vi "Power Qualtiy - 1.vi"() -> ()   [LabVIEW 2015]
uses:
  <vilib>/addons/Electrical Power/PQ/NI_EP_Power Quality.lvlib
  <vilib>/addons/Electrical Power/PQ/Aggregation/Custom Aggregation (DBL).vi
  <vilib>/addons/Electrical Power/PQ/Power_Energy/Power Values (Single Line).vi
  <vilib>/addons/Electrical Power/Basic/NI_EP_Basic.lvlib
  <vilib>/addons/Electrical Power/Basic/Measurement/Fundamental Vector (1 Channel).vi
  <vilib>/addons/Electrical Power/PQ/Common/Classes/System Info/EP System Info.lvclass
  <vilib>/addons/Electrical Power/PQ/Common/Controls/ep_AI Data Channel.ctl
  <vilib>/addons/Electrical Power/PQ/Common/Controls/ep_Aggregation Settings.ctl
  <vilib>/addons/Electrical Power/PQ/Common/Controls/ep_Event Type.ctl
  <vilib>/addons/Electrical Power/PQ/Common/Controls/ep_Phase.ctl
panel:
  out "system info out":refnum<class "EP System Info.lvclass">
  out "Pinst (Voltage Flicker Values)":waveform(dbl)[](array[waveform])
  out "rapid voltage changes events":T2(array[cluster])
  out "voltage flags":bool[](array[boolean])
  out "voltage events":T4(array[cluster])
  in  "events settings":T5={"swell threshold [%]"=110.0, "dip threshold [%]"=90.0, "interruption threshold [%]"=1.0, "hysteresis [%]"=2.0}
  out "THD [%]":dbl[](array[numeric])
  out "energy values":T6
  out "total power values":T7
  out "aggregated data timestamp":timestamp
  out "aggregated maximum value":dbl
  out "aggregated averaged/RMS value":dbl
  out "aggregated minimum value":dbl
  in  "data timestamp":timestamp
  in  "aggregation settings":T8={"interval"=1, "interval unit"=enum."Runs", "synchronization of intervals"=enum."Not synchronized", "algorithm"=enum."Average"}
  out "spectra":T10(array[cluster])
  # "System Settings"
  # "Power & Energy"
  # "Voltage"
  # "Current"
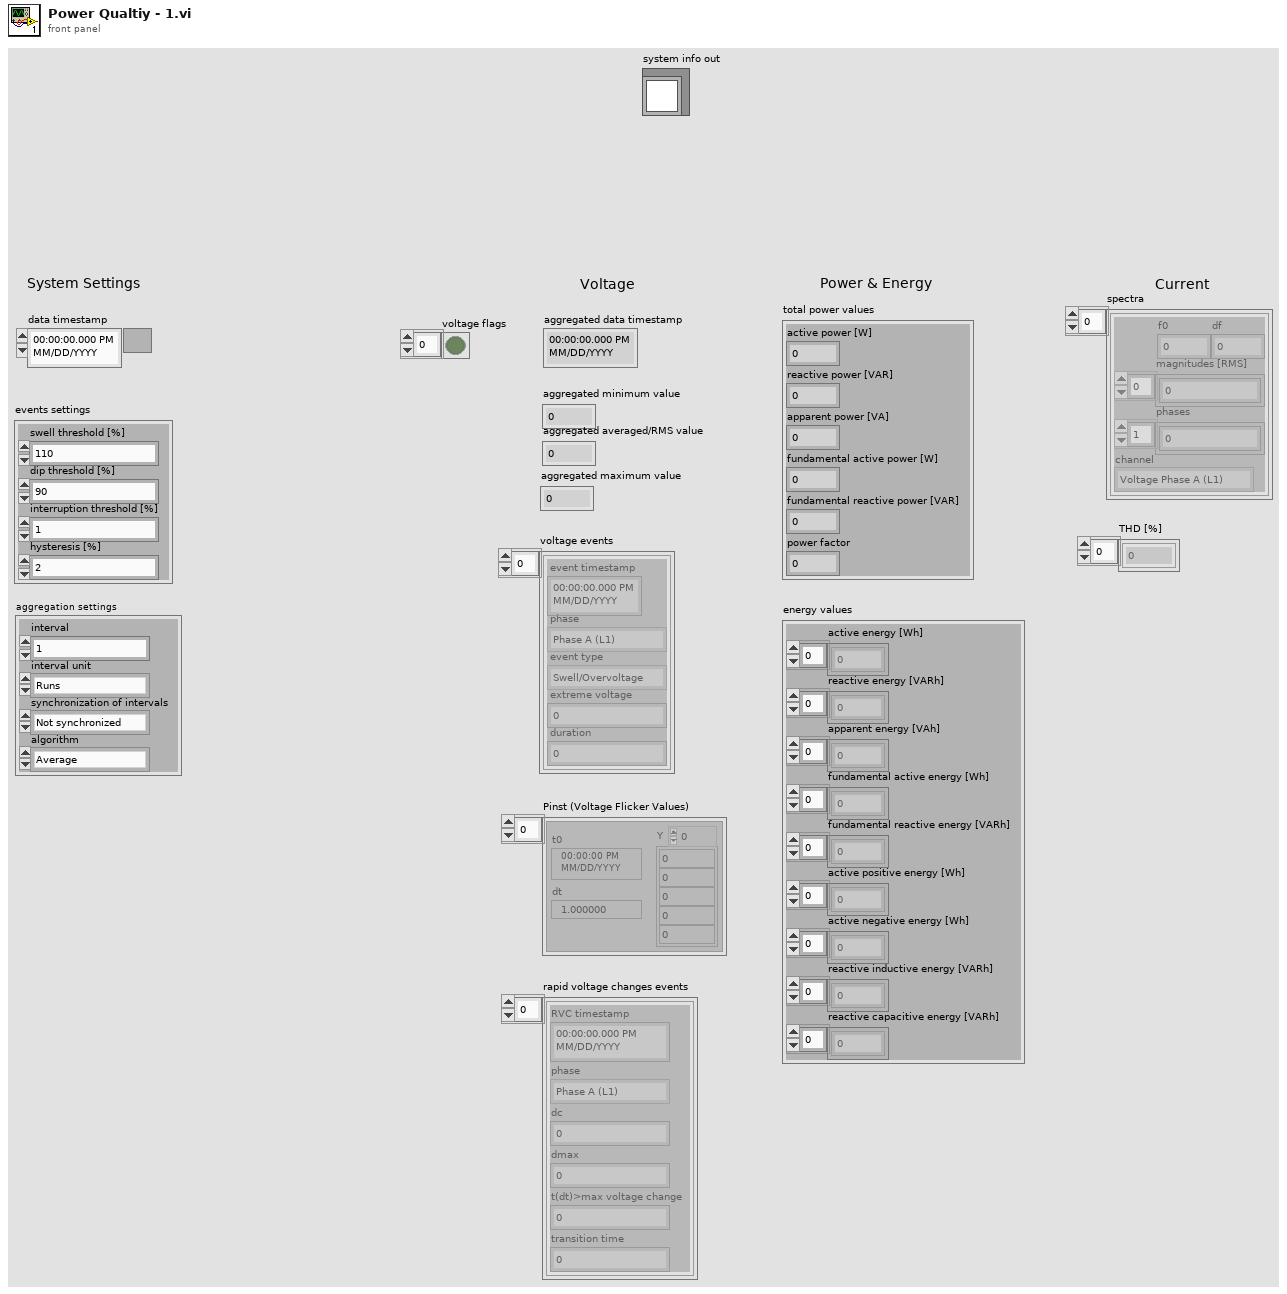
[diagram p1: front panel]
types:
  T1 = typedef "NI_EP_Power Quality.lvlib/ep_Phase.ctl" = enum16{"Phase A (L1)", "Phase B (L2)", "Phase C (L3)", "Phase N", "~3 Phases"}
  T2 = cluster{"RVC timestamp":timestamp, "phase":T1, "dc":dbl, "dmax":dbl, "t(dt)>max voltage change":dbl, "transition time":dbl}[]
  T3 = typedef "NI_EP_Power Quality.lvlib/ep_Event Type.ctl" = enum16{"Swell/Overvoltage", "Dip/Undervoltage", "Interruption"}
  T4 = cluster{"event timestamp":timestamp, "phase":T1, "event type":T3, "extreme voltage":dbl, "duration":dbl}[]
  T5 = cluster{"swell threshold [%]":dbl, "dip threshold [%]":dbl, "interruption threshold [%]":dbl, "hysteresis [%]":dbl}
  T6 = cluster{"active energy [Wh]":dbl[], "reactive energy [VARh]":dbl[], "apparent energy [VAh]":dbl[], "fundamental active energy [Wh]":dbl[], "fundamental reactive energy [VARh]":dbl[], "active positive energy [Wh]":dbl[], "active negative energy [Wh]":dbl[], "reactive inductive energy [VARh]":dbl[], "reactive capacitive energy [VARh]":dbl[]}
  T7 = cluster{"active power [W]":dbl, "reactive power [VAR]":dbl, "apparent power [VA]":dbl, "fundamental active power [W]":dbl, "fundamental reactive power [VAR]":dbl, "power factor":dbl}
  T8 = typedef "NI_EP_Power Quality.lvlib/ep_Aggregation Settings.ctl" = cluster{"interval":u32, "interval unit":enum16{"Runs", "Seconds", "Minutes", "Hours", "Days", "Weeks"}, "synchronization of intervals":enum16{"Not synchronized", "Interval rounded"}, "algorithm":enum16{"Average", "RMS"}}
  T9 = typedef "NI_EP_Power Quality.lvlib/ep_AI Data Channel.ctl" = enum16{"Voltage Phase A (L1)", "Voltage Phase B (L2)", "Voltage Phase C (L3)", "Voltage Phase N (Neutral)", "Current Phase A (L1)", "Current Phase B (L2)", "Current Phase C (L3)", "Current Phase N (Neutral)"}
  T10 = cluster{"f0":dbl, "df":dbl, "magnitudes [RMS]":dbl[], "phases":dbl[], "channel":T9}[]
  T11 = cluster{"timestamps":timestamp[], "RMS values":dbl[]}[]
  T12 = cluster{"active power [W]":dbl[], "reactive power [VAR]":dbl[], "apparent power [VA]":dbl[], "fundamental active power [W]":dbl[], "fundamental reactive power [VAR]":dbl[], "cosine":dbl[], "power factor":dbl[]}
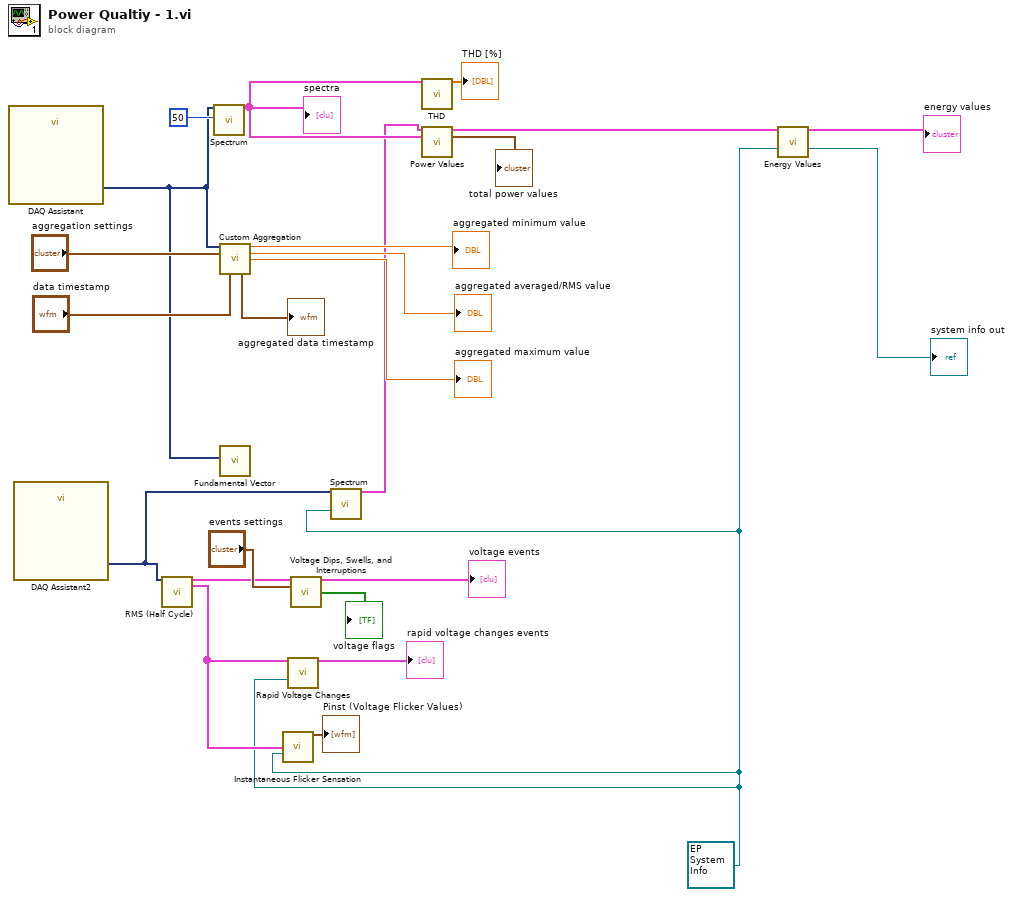
[diagram p0: block diagram]
diagram:
  w1 = refnum<class "EP System Info.lvclass"> refnum ("system info in")
  n1 = call "DAQ Assistant"() -> ("data"=w14:dynamicdata)  [unwired: 17 in, 2 out]
  n2 = call "DAQ Assistant2"() -> ("data"=w4:dynamicdata)  [unwired: 17 in, 2 out]
  n3 = call <vilib>:"RMS (Half Cycle).vi"("waveforms"=w4) -> ("one-cycle RMS"=w5:T11, "half-cycle RMS"=w7:T11)  [unwired: 11 in, 2 out]
  n4 = call <vilib>:"Spectrum.vi"("waveforms"=w14, "maximum harmonic order (50)"=u16 50) -> ("spectra"=w13:T10)  [unwired: 11 in, 2 out]
  "spectra" <- w13
  n5 = call-poly <vilib>:"Custom Aggregation.vi"("data in"=w14, "aggregation settings"="aggregation settings", "data timestamp"="data timestamp") -> ("aggregated minimum value"=→"aggregated minimum value":dbl, "aggregated averaged/RMS value"=→"aggregated averaged/RMS value":dbl, "aggregated maximum value"=→"aggregated maximum value":dbl, "aggregated data timestamp"=→"aggregated data timestamp":timestamp)  [unwired: 6 in, 3 out]
  n6 = call-poly <vilib>:"Fundamental Vector.vi"("current waveform"=w14) -> ()  [unwired: 7 in, 4 out]
  n7 = call <vilib>:"Instantaneous Flicker Sensation.vi"("half-cycle voltage RMS"=w7, "system info in"=w1) -> ("Pinst"=→"Pinst (Voltage Flicker Values)":waveform(dbl)[])  [unwired: 11 in, 2 out]
  n8 = call <vilib>:"Rapid Voltage Changes.vi"("half-cycle voltage RMS"=w7, "system info in"=w1) -> ("rapid voltage changes events"=→"rapid voltage changes events":T2)  [unwired: 11 in, 2 out]
  n9 = call <vilib>:"Voltage Dips, Swells, and Interruptions.vi"("one-cycle voltage RMS"=w5, "events settings"="events settings") -> ("voltage events"=→"voltage events":T4, "voltage flags"=→"voltage flags":bool[])  [unwired: 10 in, 2 out]
  n10 = call <vilib>:"Spectrum.vi"("waveforms"=w4, "system info in"=w1) -> ("spectra"=w3:T10)  [unwired: 11 in, 2 out]
  n11 = call <vilib>:"THD.vi"("spectra"=w13) -> ("THD [%]"=→"THD [%]":dbl[])  [unwired: 12 in, 2 out]
  n12 = call-poly <vilib>:"Power Values.vi"("phase voltage spectra"=w3, "current spectra"=w13) -> ("power values"=w17:T12, "total power values"=→"total power values":T7)  [unwired: 10 in, 2 out]
  n13 = call <vilib>:"Energy Values.vi"("power values"=w17, "system info in"=w1) -> ("energy values"=→"energy values":T6, "system info out"=→"system info out":refnum<class "EP System Info.lvclass">)  [unwired: 10 in, 2 out]
